vi "JoystickAdjustSetpoint.vi"(5 "MaxGantryIncrement":dbl, 7 "MaxLiftIncrement":dbl, 9 "PrevGantrySetpoint":dbl, 10 "PrevLiftSetpoint":dbl, 11 "Axes":dbl[](array[numeric])) -> (2 "NewGantrySetpoint":dbl, 3 "NewLiftSetpoint":dbl)   [LabVIEW 2014]
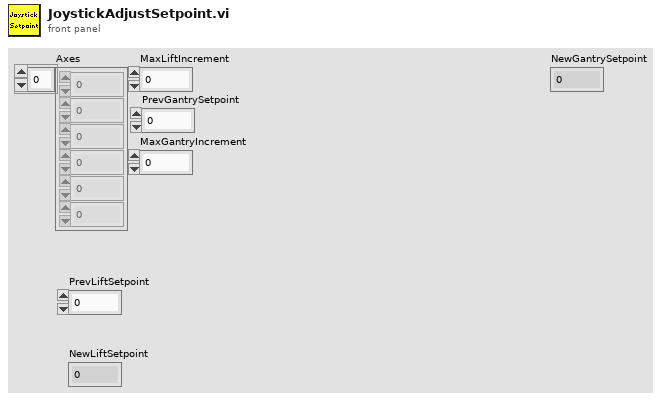
[diagram p1: front panel]
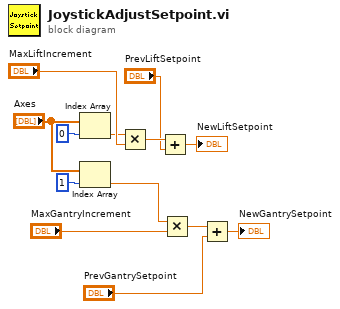
[diagram p0: block diagram]
diagram:
  n1 = Index Array(array="Axes", index=0) -> (element=w9:dbl)
  n2 = Index Array(array="Axes", index=1) -> (element=w4:dbl)
  n3 = Multiply(x=w9, y="MaxLiftIncrement") -> (x*y=w8:dbl)
  n4 = Add(x=w8, y="PrevLiftSetpoint") -> (x+y=→"NewLiftSetpoint":dbl)
  n5 = Multiply(x=w4, y="MaxGantryIncrement") -> (x*y=w5:dbl)
  n6 = Add(x=w5, y="PrevGantrySetpoint") -> (x+y=→"NewGantrySetpoint":dbl)
